vi "Test Returns Section Added.vi"(11 "Test Case In":refnum<class "Diff Tool Test.lvclass">) -> (0 "error out":errorcluster, 3 "Test Case Out":refnum<class "Diff Tool Test.lvclass">)   [LabVIEW 2020, in "Diff Tool Test.lvclass"]
uses:
  Diff Tool Test.lvclass
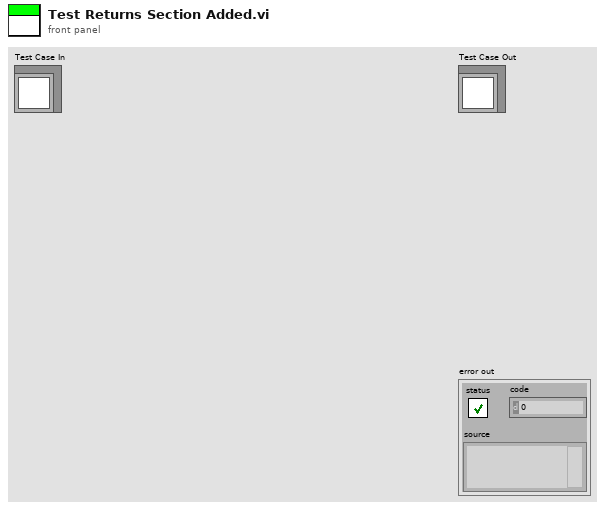
[diagram p1: front panel]
types:
  T1 = cluster{"Selection Start":u32, "Selection End":u32, "Type":enum16{"added", "missing"}}
  T2 = cluster{"Selection Start":u32, "Selection End":u32, "Type":enum16{"added", "missing"}}[]
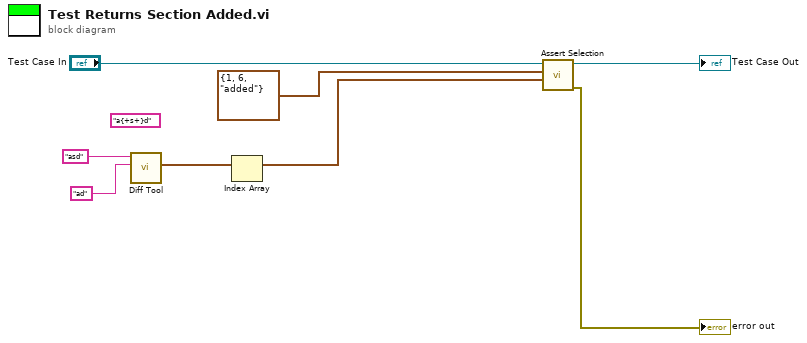
[diagram p0: block diagram]
diagram:
  (unwired) "a{+s+}d" ("Reference")
  n1 = call "Diff Tool.vi"("Reference"="ad", "Target"="asd") -> ("Highlights"=w3:T2)  [unwired: 8 in, 1 out]
  n2 = Index Array(array=w3) -> (element=w2:T1)  [unwired: 1 in]
  n3 = call "Assert Selection.vi"("Actual"=w2, "Expected"=T1 {"Selection Start"=1, "Selection End"=6, "Type"=enum."added"}, "Added Section Finder Test In"="Test Case In") -> ("error out"=→"error out":errorcluster, "Added Section Finder Test Out"=→"Test Case Out":refnum<class "Diff Tool Test.lvclass">)  [unwired: 7 in]
